vi "Inverse Kinematics.vi"(7 "armID":i32=1, 8 "z":dbl, 9 "y":dbl, 10 "x":dbl, 11 "toolInsertionOffset":dbl=-54.76) -> (1 "j3":dbl, 2 "j2":dbl, 3 "j1":dbl, 5 "return type":i32)   [LabVIEW 2016]
uses:
  Subsystems/Global Variables.vi
  RobotKinematicsDLL.dll
panel:
  out "KINEMATICS_RET_SOLUTION_BEYOND_LIMIT":bool
  out "KINEMATICS_RET_NO_SOLUTION":bool
  out "KINEMATICS_RET_WRONG_ARM_ID":bool
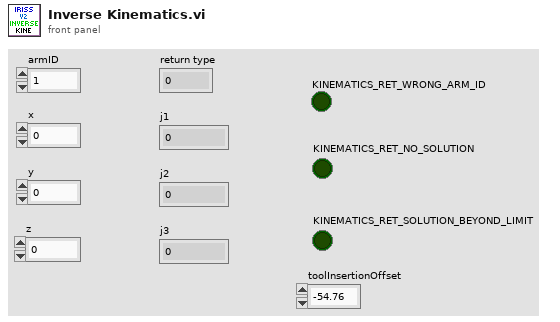
[diagram p1: front panel]
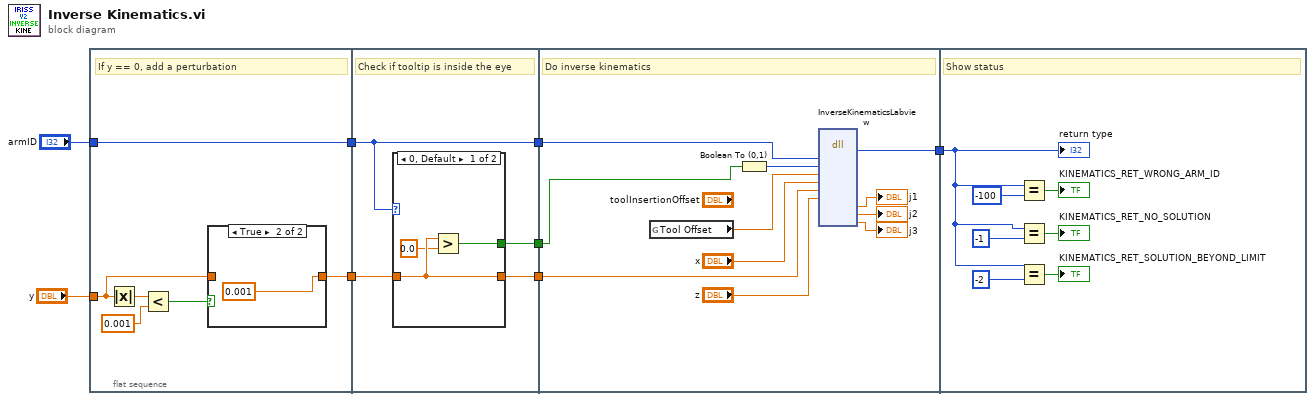
[diagram p0: block diagram]
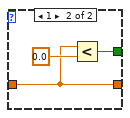
[diagram p3: hidden frame]
diagram:
  n1 = flat-sequence {
    tunnel: "y" -> [w9]
    tunnel: "armID" -> [w14]
    tunnel: [w14] -> w4
    tunnel: [w13] -> w3
    tunnel: [w20] -> w7
    tunnel: [w18] -> w5
    tunnel: w4 -> [w20]
    tunnel: w3 -> [w19]
    tunnel: [w17] -> w2
    tunnel: w7 -> [w30]
    tunnel: w5 -> [w29]
    tunnel: w2 -> [w27]
    tunnel: [w28] -> w1
    tunnel: w1 -> [w38]
    frame #0 {
      # "If y == 0, add a perturbation"
      n2 = Absolute Value(x=w9) -> (abs(x)=w12:dbl)
      n3 = Less?(x=w12, y=0.001) -> (x < y?=w10:bool)
      n4 = case shown="True" w10 {
        tunnel: w9 -> [w15 _]
        tunnel: [w15 0.001 ("y")] -> w13
        frame False {
        }
        frame True {
        }
      }
    }
    frame #1 {
      # "Check if tooltip is inside the eye"
      n5 = case shown="0, Default" w20 {
        tunnel: w19 -> [w23 w24]
        tunnel: [w23 w24] -> w18
        tunnel: [w21 w25] -> w17
        frame 0, Default {
          n6 = Greater?(x=w23, y=0.0) -> (0:w21:bool)
        }
        frame 1 {
          n7 = Less?(x=w24, y=0.0) -> (x < y?=w25:bool)
        }
      }
    }
    frame #2 {
      # "Do inverse kinematics"
      n8 = global read "Global Variables.vi" "Tool Offset"() -> (w37:dbl)
      n9 = Boolean To (0,1)(Boolean=w27) -> (0, 1=w36:i16)
      n10 = dll-call lib="D:/Kevin/IRISS V2 dev/Host Demo/Functions/RobotKinematicsDLL.dll" fn="InverseKinematicsLabview"("id"=w30, "isToolInsideEye"=w36, "toolInsertionOffset"=w37, "x"="x", "y"=w29, "z"="z") -> ("return type"=w28:i32, "j1"=→"j1":dbl, "j2"=→"j2":dbl, "j3"=→"j3":dbl)  [unwired: 12 in, 2 out]
    }
    frame #3 {
      # "Show status"
      n11 = Equal?(x=w38, y=-100) -> (x = y?=→"KINEMATICS_RET_WRONG_ARM_ID":bool)
      n12 = Equal?(x=w38, y=-1) -> (x = y?=→"KINEMATICS_RET_NO_SOLUTION":bool)
      n13 = Equal?(x=w38, y=-2) -> (x = y?=→"KINEMATICS_RET_SOLUTION_BEYOND_LIMIT":bool)
      "return type" <- w38
    }
  }
